vi "property_write_read.vi"(10 "value":u32, 11 "Digital in":refnum<vi>) -> (3 "result":u32)   [LabVIEW 2020]
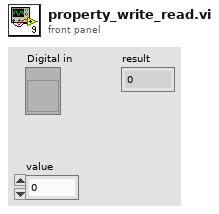
[diagram p1: front panel]
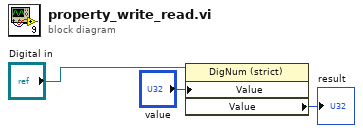
[diagram p0: block diagram]
diagram:
  n1 = property class="DigNum (strict)"(reference="Digital in", "Value"="value") -> ("Value"=→"result":u32)  [unwired: 1 in, 2 out]
